vi "GetVoiceData.vi"(8 "error in":errorcluster, 10 "filePath":path, 11 "Path In":path) -> (0 "error out":errorcluster, 1 "Fs":dbl, 2 "voiceData":dbl[](array[numeric]), 3 "Path Out":path)   [LabVIEW 2015]
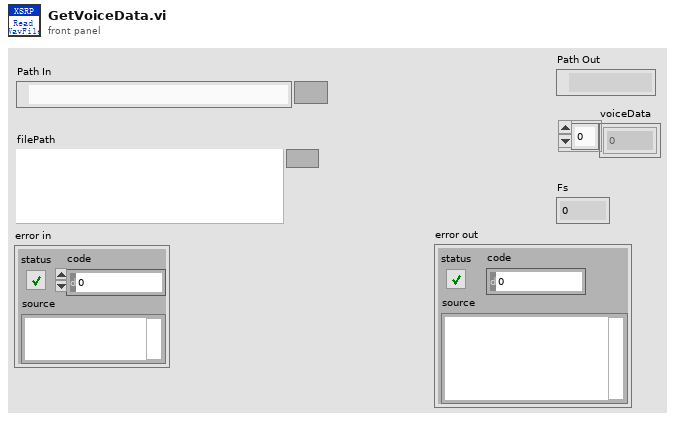
[diagram p1: front panel]
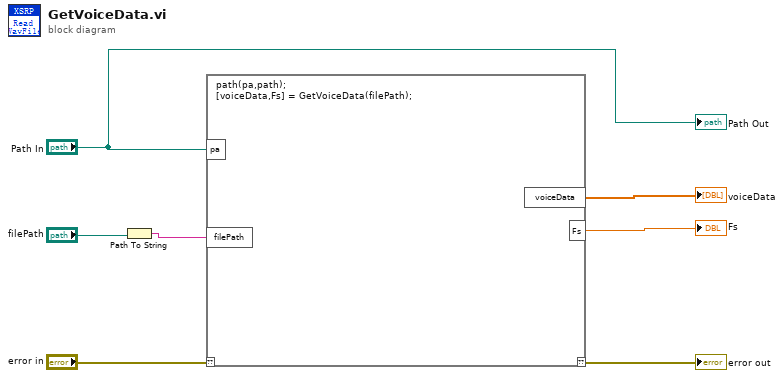
[diagram p0: block diagram]
diagram:
  n1 = Path To String(path="filePath") -> (string=w1:string)
  n2 = script code="path(pa,path);\n[voiceData,Fs] = GetVoiceData(filePath);"("??"="error in", "pa"="Path In", "filePath"=w1) -> ("??"=→"error out":errorcluster, "voiceData"=→"voiceData":dbl[], "Fs"=→"Fs":dbl)
  "Path Out" <- "Path In"
